vi "CODMN外部API.vi"() -> ()   [LabVIEW 2016, in "斯坦道CODMn.lvlib"]
panel:
  out "手动启动CODMn":bool
  in  "CODMn外围API":T1
  in  "自动切换量程":bool=TRUE
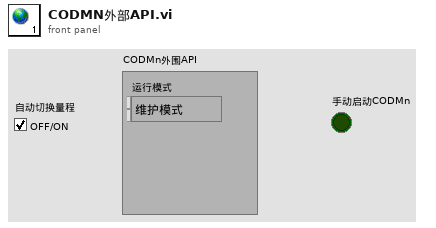
[diagram p1: front panel]
types:
  T1 = cluster{"运行模式":enum16{"维护模式", "常规模式", "应急模式", "质控模式"}}
diagram:
